vi "Stream_IncrementBlock.vi"(8 "error in (no error)":errorcluster, 9 "last block":bool, 10 "stream Id in":string, 11 "streams in":variant) -> (0 "error out":errorcluster, 1 "next block":i32, 2 "stream ID out":string, 3 "streams out":variant, 5 "open stream":bool)   [LabVIEW 2017, in "FileManager.lvlib"]
uses:
  <vilib>/addons/InsightCM/Devices/Shared/Common/FileManager/FileManager.lvlib
  <vilib>/addons/InsightCM/Devices/Shared/Common/FileManager/controls/StreamState.ctl
panel:
  # "Deprecated - used for TDMS and TDMS in memory"
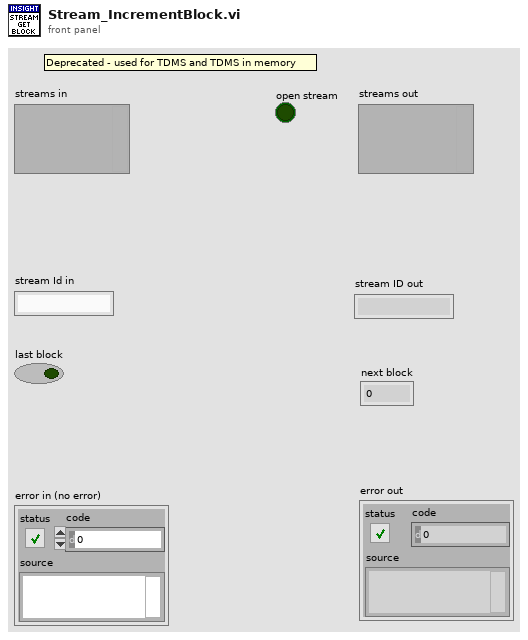
[diagram p1: front panel]
types:
  T1 = typedef "FileManager.lvlib/StreamState.ctl" = cluster{"DataGroup":string, "Stream Id":string, "LastBlock":bool, "TotalBlocks":i32, "BlocksSent":i32, "Device":string}
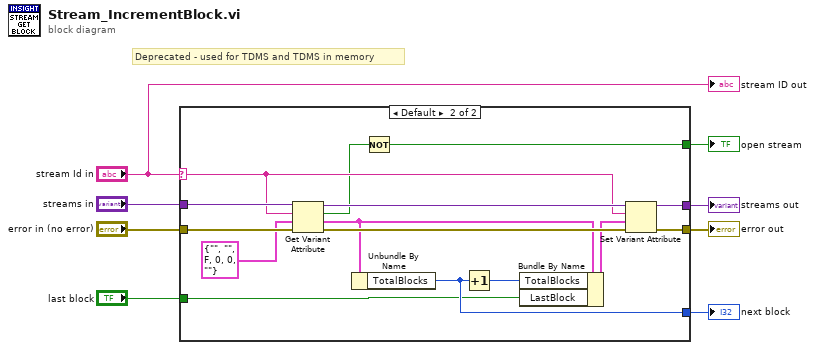
[diagram p0: block diagram]
diagram:
  # "Deprecated - used for TDMS and TDMS in memory"
  n1 = case shown="Default" "stream Id in" {
    selector: "stream Id in" -> [_ w13]
    tunnel: "error in (no error)" -> [w10 w25]
    tunnel: "streams in" -> [w9 w24]
    tunnel: [w10 w22] -> w6
    tunnel: [_ w19] -> w5
    tunnel: [w9 w15] -> w4
    tunnel: "last block" -> [_ w14]
    tunnel: [_ w11] -> w1
    frame "" {
    }
    frame Default {
      n2 = Get Variant Attribute(Variant=w24, name=w13, default value (empty Variant)=T1 {"DataGroup"="", "Stream Id"="", "LastBlock"=FALSE, "TotalBlocks"=0, "BlocksSent"=0, "Device"=""} ("Stream"), error in=w25) -> (duplicate Variant=w16:variant, found=w12:bool, value=w20:T1, error out=w23:errorcluster)
      n3 = Unbundle By Name(w20) -> ("TotalBlocks"=w19:i32)
      n4 = Not(x=w12) -> (.not. x?=w11:bool)
      n5 = Increment(x=w19) -> (x+1=w18:i32)
      n6 = Bundle By Name(cluster=w20, "TotalBlocks"=w18, "LastBlock"=w14) -> (w17:T1)
      n7 = Set Variant Attribute(Variant=w16, name=w13, value=w17, error in=w23) -> (Variant out=w15:variant, error out=w22:errorcluster)  [unwired: 1 out]
    }
  }
  "streams out" <- w4
  "next block" <- w5
  "error out" <- w6
  "open stream" <- w1
  "stream ID out" <- "stream Id in"
